vi "visa_close.vi"() -> ()   [LabVIEW 2012]
panel:
  out "error out":errorcluster caption="エラー出力"
  in  "VISAリソース名":refnum<visa-resource-name>="COM5"
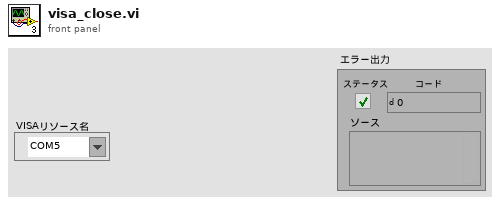
[diagram p1: front panel]
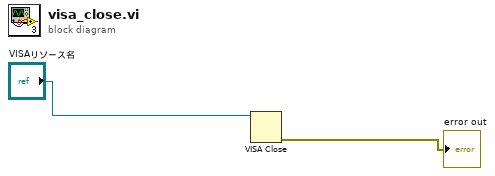
[diagram p0: block diagram]
diagram:
  n1 = VISA Close(VISA resource name="VISAリソース名") -> (error out=→"error out":errorcluster)  [unwired: 1 in]
